vi "Configure Power Offset.vi"(8 "error in (no error)":errorcluster, 10 "Power Offset":dbl, 11 "U2000 in":refnum<class "U2000.lvclass">) -> (0 "error out":errorcluster, 3 "U2000 out":refnum<class "U2000.lvclass">)   [LabVIEW 2020, in "U2000.lvclass"]
uses:
  U2000.lvclass
  C:/Sandbox/RF Bench/Source Code/WiSpry Test Framework/Instruments/Instrument.lvclass
  Instrument.lvclass/Instrument.ctl
  <instrlib>/Agilent U2000 Series/Agilent U2000 Series.lvlib
  Instrument.lvclass
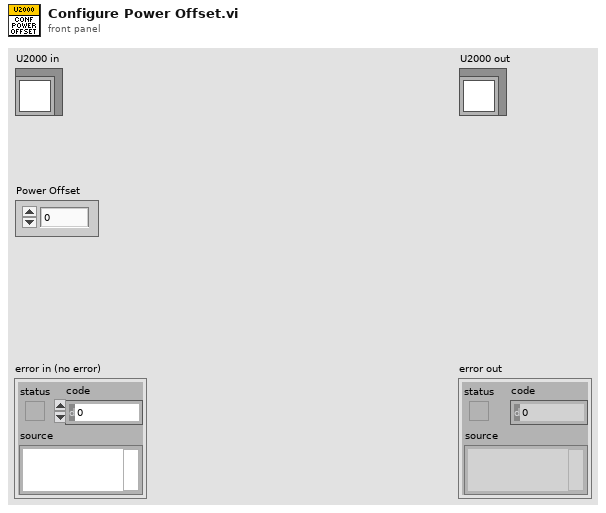
[diagram p1: front panel]
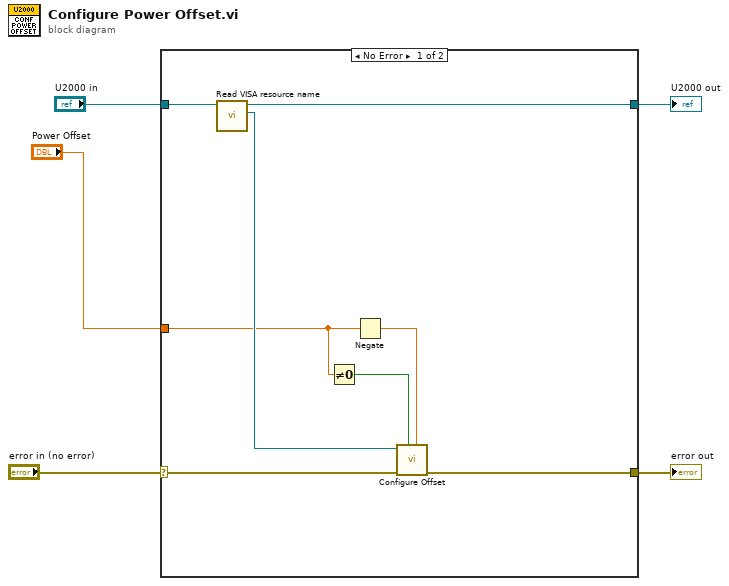
[diagram p0: block diagram]
diagram:
  n1 = case shown="No Error" "error in (no error)" {
    selector: "error in (no error)" -> [w13 w15]
    tunnel: [w12 w15] -> w4
    tunnel: "U2000 in" -> [w11 w14]
    tunnel: [w10 w14] -> w2
    tunnel: "Power Offset" -> [w7 _]
    frame No Error {
      n2 = call "Read VISA resource name.vi"("Instrument in"=w11) -> ("VISA resource name"=w9:refnum<visa-resource-name>, "Instrument out"=w10:refnum<class "U2000.lvclass">)  [unwired: 9 in]
      n3 = Not Equal To 0?(x=w7) -> (x != 0?=w8:bool)
      n4 = Negate(x=w7) -> (-x=w6:dbl)
      n5 = call <instrlib>:"Configure Offset.vi"("Offset Value (0 dB)"=w6, "Enable Offset (F: Disable)"=w8, "error in (no error)"=w13, "VISA resource name"=w9) -> ("error out"=w12:errorcluster)  [unwired: 6 in, 1 out]
    }
    frame Error {
    }
  }
  "error out" <- w4
  "U2000 out" <- w2
